vi "Ger All Station Alias Name.vi"(11 "Stations":cluster{"Stations":string, "alias":string}[](array[cluster])) -> (3 "Array":string[](array[string]))   [LabVIEW 2014]
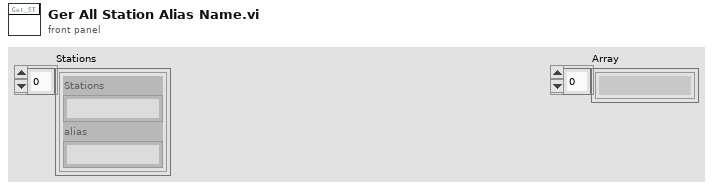
[diagram p1: front panel]
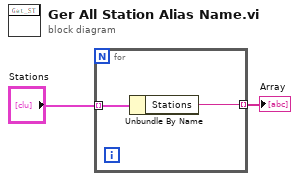
[diagram p0: block diagram]
diagram:
  n1 = for {
    tunnel: "Stations" -> [w4] mode=indexing
    tunnel: [w3] -> w1 mode=indexing
    n2 = Unbundle By Name(w4) -> ("Stations"=w3:string)
  }
  "Array" <- w1
